vi "Set XY Graph Y Range.vi"(8 "error in (no error)":errorcluster, 9 "Maximum [1]":dbl=1.0, 10 "Minimum [0]":dbl, 11 "graph_utilities in":refnum<class "graph_utilities.lvclass">) -> (0 "error out":errorcluster, 3 "graph_utilities out":refnum<class "graph_utilities.lvclass">)   [LabVIEW 2016, in "graph_utilities.lvclass"]
doc: "Set the X Range (<b>Minimum</b> and <b>Maximum</b>) of the XY Graph."
uses:
  graph_utilities.lvclass
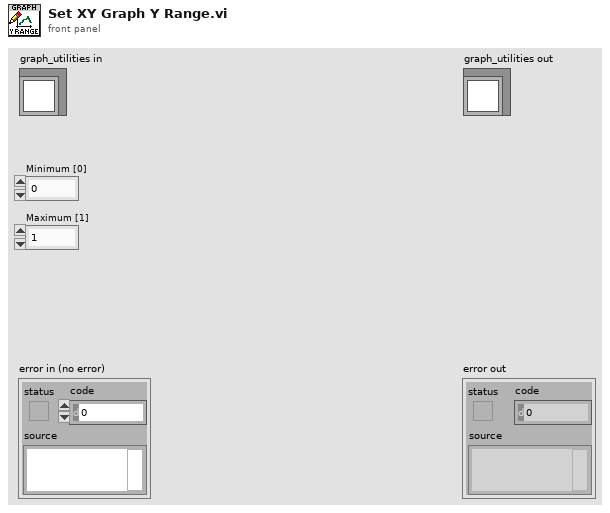
[diagram p1: front panel]
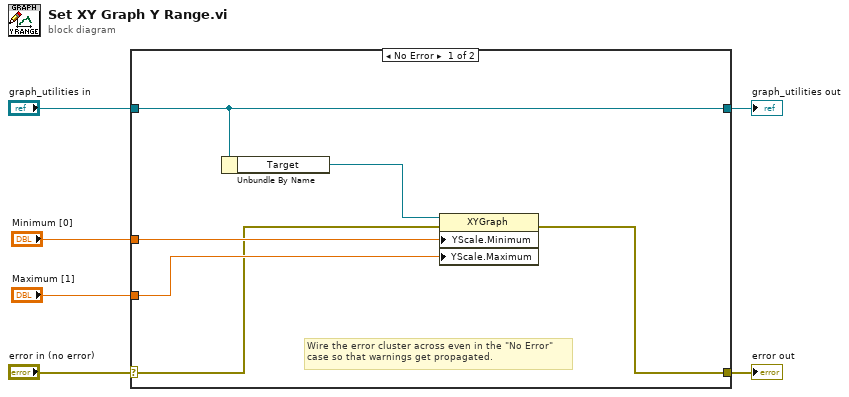
[diagram p0: block diagram]
diagram:
  n1 = case shown="No Error" "error in (no error)" {
    selector: "error in (no error)" -> [w8 w14]
    tunnel: [w7 w14] -> w5
    tunnel: [w12 w13] -> w3
    tunnel: "graph_utilities in" -> [w12 w13]
    tunnel: "Minimum [0]" -> [w10 _]
    tunnel: "Maximum [1]" -> [w9 _]
    frame No Error {
      # "Wire the error cluster across even in the \"No Error\"\ncase so that warnings get propagated."
      n2 = Unbundle By Name(w12) -> ("Target"=w11:refnum<vi>)
      n3 = property on="Property Node" class="XYGraph"(reference=w11, error in=w8, "YScale.Minimum"=w10, "YScale.Maximum"=w9) -> (error out=w7:errorcluster)  [unwired: 1 out]
    }
    frame Error {
    }
  }
  "error out" <- w5
  "graph_utilities out" <- w3
